vi "Validate.vi"(0 "ControlDoBase in":refnum<class "ControlActionBase.lvclass">, 11 "error in (no error)":errorcluster) -> (4 "ControlDoBase out":refnum<class "ControlActionBase.lvclass">, 15 "error out":errorcluster)   [LabVIEW 2016, in "ControlActionBase.lvclass"]
uses:
  ControlActionBase.lvclass
  ControlActionBase.lvclass/ControlActionBase.ctl
  <vilib>/Utility/error.llb/Error Cluster From Error Code.vi
  <vilib>/ErrorRing/Error Ring.xnode
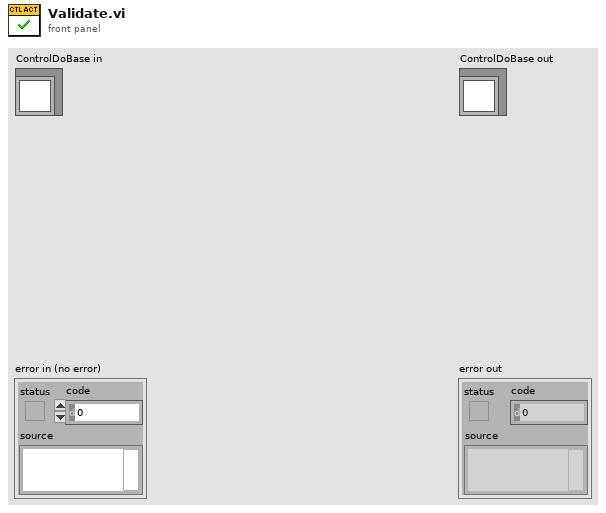
[diagram p1: front panel]
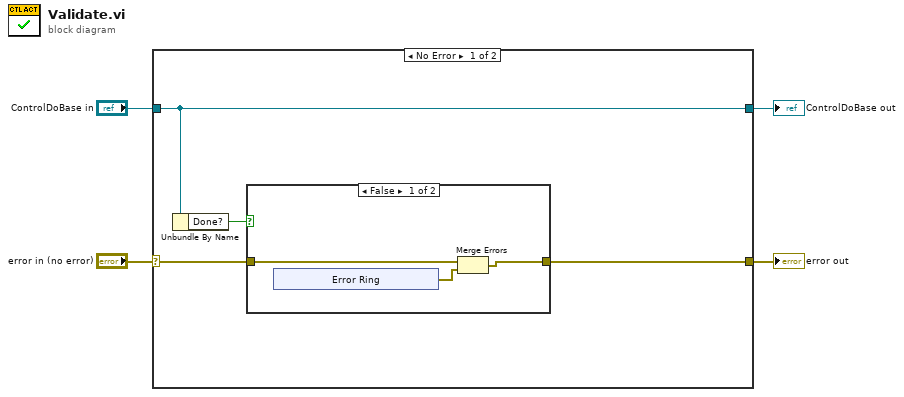
[diagram p0: block diagram]
diagram:
  n1 = case shown="No Error" "error in (no error)" {
    selector: "error in (no error)" -> [w8 w19]
    tunnel: [w6 w19] -> w3
    tunnel: [w7 w18] -> w1
    tunnel: "ControlDoBase in" -> [w7 w18]
    frame No Error {
      n2 = Unbundle By Name(w7) -> ("Done?"=w5:bool)
      n3 = case shown="False" w5 {
        tunnel: w8 -> [w11 w17]
        tunnel: [w10 w17] -> w6
        frame False {
          n4 = xnode "Error Ring"() -> ("error out"=w9:errorcluster)
          n5 = Merge Errors(w11, w9) -> (w10:errorcluster)
        }
        frame True {
        }
      }
    }
    frame Error {
    }
  }
  "error out" <- w3
  "ControlDoBase out" <- w1
